vi "Main.vi"() -> ()   [LabVIEW 2019, in "Chat Window.lvlib"]
doc: "This template is based off of the Queued Message Handler design pattern and the Queued Message Handler project template that ships with LabVIEW.\n\nThe main difference is that the queue is private to this module and communication between modules is performed via Broadcast and Request events.\n\nRequest events are wrapped in public API methods and are handled in the Event Handling Loop (EHL) of this VI. Any module can register for Broadcast events sent by this module. The EHL generates messages based on user interface actions.\n\nThe Message Handling Loop (MHL) processes messages generated by the EHL, or by other messages. The messages are string values, so new messages can be added easily to the Message Cases case structure in the MHL. Each message cluster can also provide an optional value for Message Data, which is a variant that can be converted to whatever message-specific data is required.\n_____\nBased on Delacor QMH Project Template 4.2.1.64."
uses:
  Chat Window.lvlib
  <vilib>/Delacor/Delacor QMH/Libraries/Cloneable Module Admin_class/Delacor_lib_QMH_Cloneable Module Admin.lvclass
  C:/Program Files (x86)/National Instruments/LabVIEW 2019/vi.lib/Delacor/Delacor QMH/Libraries/Module Admin_class/Delacor_lib_QMH_Module Admin.lvclass
  Module Data--cluster.ctl
  <vilib>/Delacor/Delacor QMH/Libraries/Message Queue_class/Delacor_lib_QMH_Message Queue.lvclass/Delacor_lib_QMH_Message Queue.ctl
  <vilib>/Delacor/Delacor QMH/Libraries/Cloneable Module Admin_class/Delacor_lib_QMH_Cloneable Module Admin.lvclass/Delacor_lib_QMH_Cloneable Module Admin.ctl
  Stop Argument--cluster.ctl
  New Message Argument--cluster.ctl
  Update Ring Argument--cluster.ctl
  <vilib>/Utility/miscctls.llb/LVPointTypeDef.ctl
  <vilib>/Delacor/Delacor QMH/Libraries/Module Admin_class/Delacor_lib_QMH_Module Admin.lvclass/Delacor_lib_QMH_Module Admin.ctl
  <vilib>/Delacor/Delacor QMH/Libraries/Message Queue_class/Delacor_lib_QMH_Enqueue Message (Single).vi
  <vilib>/Delacor/Delacor QMH/Libraries/Cloneable Module Admin_class/Delacor_lib_QMH_Get Module ID.vi
  <vilib>/Delacor/Delacor QMH/Libraries/Module Admin_class/Delacor_lib_QMH_Get External Launch.vi
  <vilib>/Utility/error.llb/Error Cluster From Error Code.vi
  <vilib>/ErrorRing/Error Ring.xnode
  <vilib>/Delacor/Delacor QMH/Libraries/Message Queue_class/Delacor_lib_QMH_Message Queue.lvclass
  Clone Registration/Clone Registration.lvlib
panel:
  in  "Chat Window Selection":i32(ring) items=["All"=-1]
  in  "Send":bool
  in  "Messages Out":string
  out "Messages In":string
  in  "Simulate MHL Error":bool
  in  "Simulate EHL Error":bool
  out "error out":errorcluster
  in  "Module Admin":refnum<class "Delacor_lib_QMH_Cloneable Module Admin.lvclass">
  out "Status":string
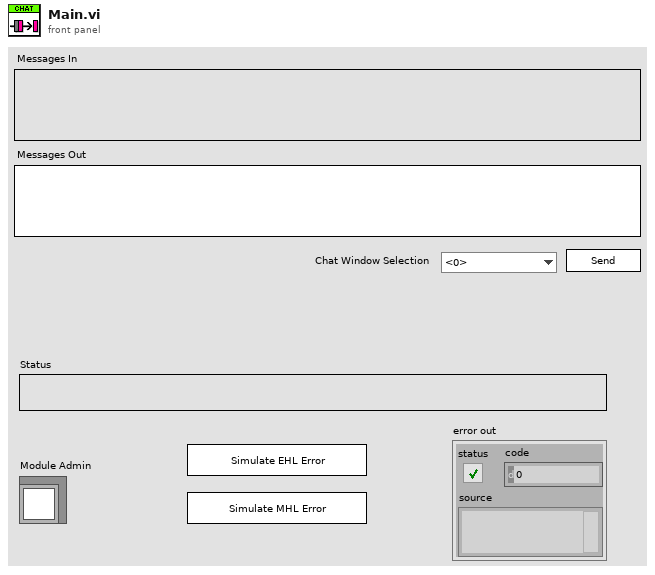
[diagram p1: front panel]
types:
  T1 = typedef "Chat Window.lvlib/Request Events--cluster.ctl" = cluster{"Stop Module":refnum<user-event>, "Show Panel":refnum<user-event>, "Hide Panel":refnum<user-event>, "Show Diagram":refnum<user-event>, "Get Module Execution Status":refnum<user-event>, "New Message":refnum<user-event>, "Update Ring":refnum<user-event>}
  T2 = typedef "Chat Window.lvlib/Module Data--cluster.ctl" = cluster{"Status":string}
  T3 = enum32{"invalid lock state", "Not Locked", "Locked (No Password)", "Password-protected"}
  T4 = typedef "Chat Window.lvlib/Stop Argument--cluster.ctl" = cluster{"Module ID":i32, "Origin":string, "Exit via Stop Module Req?":bool, "Wait for Module to stop?":bool}
  T5 = typedef "Chat Window.lvlib/New Message Argument--cluster.ctl" = cluster{"Module ID":i32, "Chat Message":string}
  T6 = typedef "Chat Window.lvlib/Update Ring Argument--cluster.ctl" = cluster{"Module ID":i32, "Boolean":bool}
  T7 = typedef "LVPointTypeDef.ctl" = cluster{"Horizontal":i16, "Vertical":i16}
  T8 = enum32{"Invalid", "Standard", "Closed", "Hidden", "Minimized", "Maximized"}
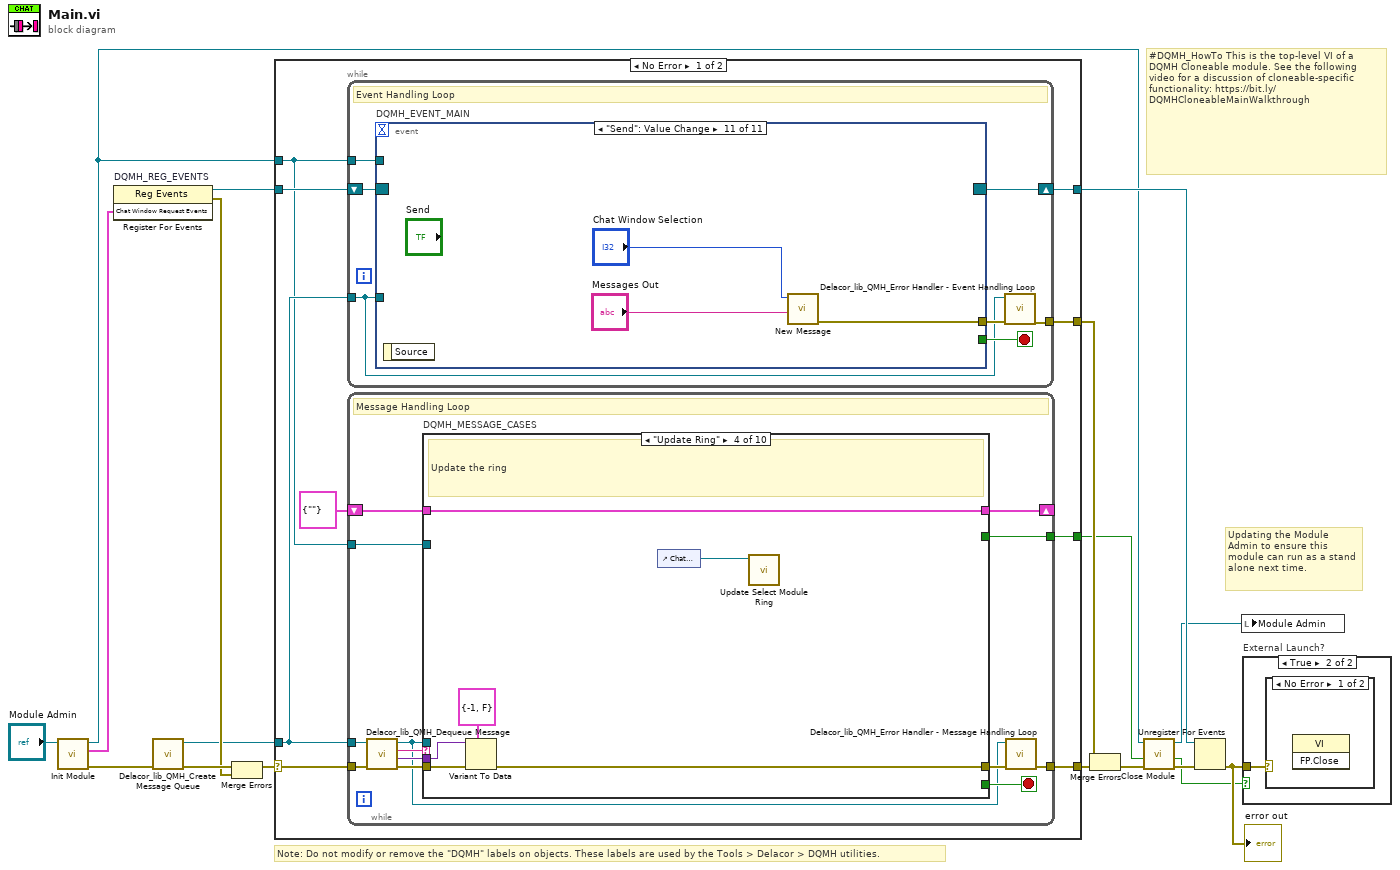
[diagram p0: block diagram]
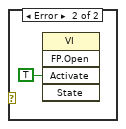
[diagram p3: hidden frame]
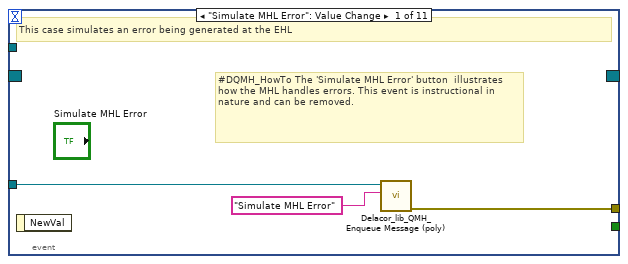
[diagram p4: hidden frame]
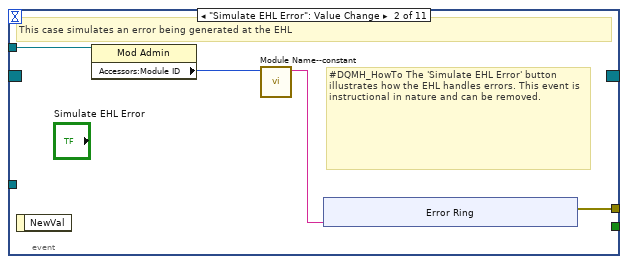
[diagram p5: hidden frame]
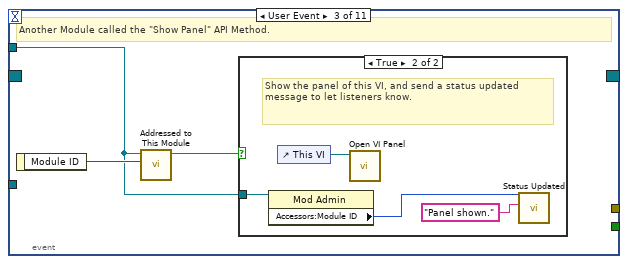
[diagram p6: hidden frame]
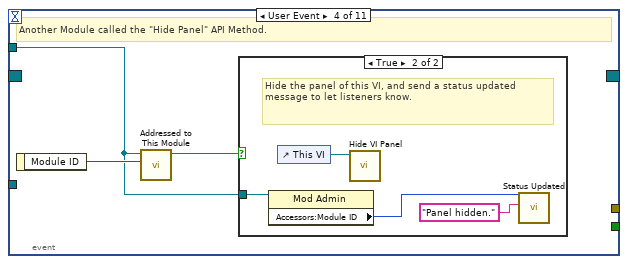
[diagram p8: hidden frame]
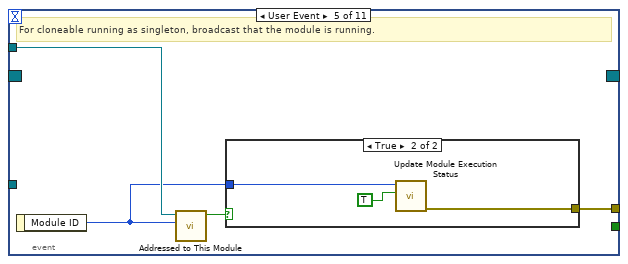
[diagram p10: hidden frame]
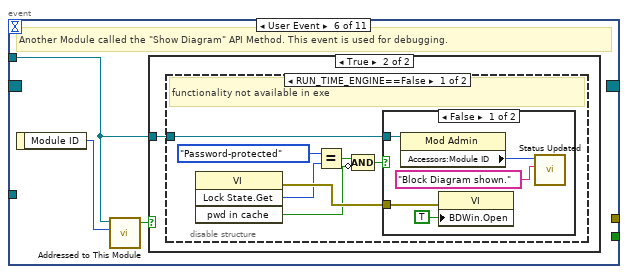
[diagram p12: hidden frame]
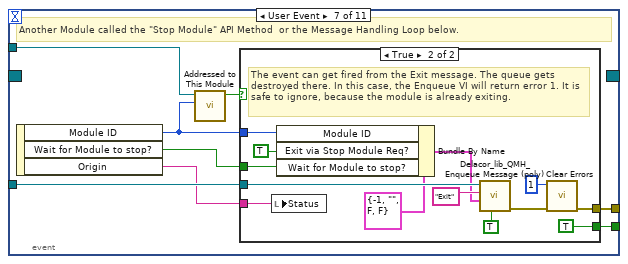
[diagram p16: hidden frame]
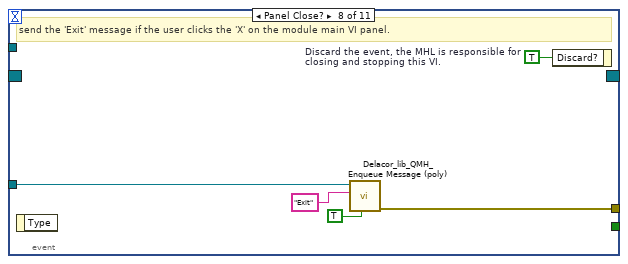
[diagram p18: hidden frame]
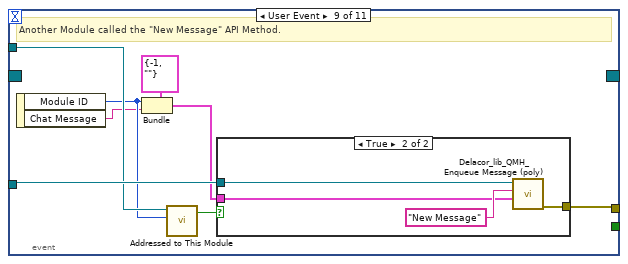
[diagram p19: hidden frame]
diagram:
  # "#DQMH_HowTo This is the top-level VI of a DQMH Cloneable module. See the following video for a discussion of cloneable-specific functionality: https://bit.ly/DQMHCloneableMainWalkthrough"
  # "Note: Do not modify or remove the \"DQMH\" labels on objects. These labels are used by the Tools > Delacor > DQMH utilities."
  # "Updating the Module Admin to ensure this module can run as a stand alone next time."
  n1 = call "Init Module.vi"("Cloneable Module Admin in"="Module Admin") -> ("error out"=w15:errorcluster, "Chat Window Request Events"=w7:T1, "Cloneable Module Admin out"=w4:refnum<class "Delacor_lib_QMH_Cloneable Module Admin.lvclass">)  [unwired: 8 in]
  n2 = register-events "DQMH_REG_EVENTS"(w7) -> (reference out=w8:refnum<event-registration>, error out=w10:errorcluster)  [unwired: 2 in]
  n3 = call <vilib>:"Delacor_lib_QMH_Create Message Queue.vi"("error in (no error)"=w15) -> ("error out"=w12:errorcluster, "Message Queue"=w6:refnum<class "Delacor_lib_QMH_Message Queue.lvclass">)  [unwired: 9 in]
  n4 = Merge Errors(w12, w10) -> (w11:errorcluster)
  n5 = case shown="No Error" w11 {
    selector: w11 -> [w25 w264]
    tunnel: [w27 w264] -> w16
    tunnel: [w24 w263] -> w9
    tunnel: w8 -> [w22 w263]
    tunnel: w6 -> [w21 _]
    tunnel: [w26 _] -> w17
    tunnel: w4 -> [w20 w259]
    tunnel: [w19 _] -> w2
    frame No Error {
      n6 = while {
        tunnel: w21 -> [w28]
        shift-right: [w31] -> w24
        shift-left: w22 -> [w32]
        tunnel: [w33] -> w26
        tunnel: w20 -> [w29]
        stop <- w30 stop-if-true
        # "Event Handling Loop"
        n7 = event "DQMH_EVENT_MAIN" shown="[10] \"Send\": Value Change" {
          selector: w32 -> [_ _ _ _ _ _ _ _ _ _ _]
          dyn-events: [_ _ _ _ _ _ _ _ _ _ _] -> w31
          timeout: _ -> [_ _ _ _ _ _ _ _ _ _ _]
          tunnel: [_ _ _ _ _ _ w89 _ _ _ _] -> w30
          tunnel: w28 -> [w36 _ _ _ _ _ w92 w109 w119 w131 _]
          tunnel: [w37 w41 _ _ w66 _ w93 w111 w112 w124 w136] -> w34
          tunnel: w29 -> [_ w40 w49 w56 w64 w70 w91 _ w117 w129 _]
          event "Simulate MHL Error": Value Change {
            # "#DQMH_HowTo The 'Simulate MHL Error' button  illustrates how the MHL handles errors. This event is instructional in nature and can be removed."
            # "This case simulates an error being generated at the EHL"
            n8 = event-data() -> ()  [unwired: 1 in, 1 out]
            n9 = call-poly <vilib>:"Delacor_lib_QMH_Enqueue Message (poly).vi"("Message"="Simulate MHL Error", "Message Queue in"=w36) -> ("error out"=w37:errorcluster)  [unwired: 8 in, 1 out]
          }
          event "Simulate EHL Error": Value Change {
            # "#DQMH_HowTo The 'Simulate EHL Error' button  illustrates how the EHL handles errors. This event is instructional in nature and can be removed."
            # "This case simulates an error being generated at the EHL"
            n10 = event-data() -> ()  [unwired: 1 in, 1 out]
            n11 = property class="Mod Admin"(reference=w40) -> ("Accessors:Module ID"=w39:i32)  [unwired: 1 in, 2 out]
            n12 = call "Module Name--constant.vi"("Module ID"=w39) -> ("Module Name"=w38:string)  [unwired: 10 in]
            n13 = xnode "Error Ring"("parameter 0"=w38) -> ("error out"=w41:errorcluster)
          }
          event User Event {
            # "Another Module called the \"Show Panel\" API Method."
            n14 = event-data() -> ("Module ID"=w50:i32)  [unwired: 1 in]
            n15 = call "Addressed to This Module.vi"("Module ID from Argument"=w50, "Module Admin"=w49) -> ("Addressed to this instance?"=w51:bool)  [unwired: 8 in, 1 out]
            n16 = case shown="True" w51 {
              tunnel: w49 -> [_ w53]
              frame False {
              }
              frame True {
                # "Show the panel of this VI, and send a status updated message to let listeners know."
                n17 = property class="Mod Admin"(reference=w53) -> ("Accessors:Module ID"=w52:i32)  [unwired: 1 in, 2 out]
                n18 = control-ref of="This VI"() -> (w55:refnum<vi>)
                n19 = call "Open VI Panel.vi"("VI"=w55) -> ()  [unwired: 10 in, 1 out]
                n20 = call "Status Updated.vi"("Status"="Panel shown." ("format string"), "Module ID"=w52) -> ()  [unwired: 9 in, 1 out]
              }
            }
          }
          event User Event {
            # "Another Module called the \"Hide Panel\" API Method."
            n21 = event-data() -> ("Module ID"=w57:i32)  [unwired: 1 in]
            n22 = call "Addressed to This Module.vi"("Module ID from Argument"=w57, "Module Admin"=w56) -> ("Addressed to this instance?"=w58:bool)  [unwired: 8 in, 1 out]
            n23 = case shown="True" w58 {
              tunnel: w56 -> [_ w60]
              frame False {
              }
              frame True {
                # "Hide the panel of this VI, and send a status updated message to let listeners know."
                n24 = property class="Mod Admin"(reference=w60) -> ("Accessors:Module ID"=w59:i32)  [unwired: 1 in, 2 out]
                n25 = control-ref of="This VI"() -> (w62:refnum<vi>)
                n26 = call "Hide VI Panel.vi"("VI"=w62) -> ()  [unwired: 10 in, 1 out]
                n27 = call "Status Updated.vi"("Status"="Panel hidden." ("format string"), "Module ID"=w59) -> ()  [unwired: 9 in, 1 out]
              }
            }
          }
          event User Event {
            # "For cloneable running as singleton, broadcast that the module is running."
            n28 = event-data() -> ("Module ID"=w63:i32)  [unwired: 1 in]
            n29 = call "Addressed to This Module.vi"("Module ID from Argument"=w63, "Module Admin"=w64) -> ("Addressed to this instance?"=w65:bool)  [unwired: 8 in, 1 out]
            n30 = case shown="True" w65 {
              tunnel: [_ w69] -> w66
              tunnel: w63 -> [_ w68]
              frame False {
              }
              frame True {
                n31 = call "Update Module Execution Status.vi"("Running?"=TRUE, "Module ID"=w68) -> ("error out"=w69:errorcluster)  [unwired: 9 in]
              }
            }
          }
          event User Event {
            # "Another Module called the \"Show Diagram\" API Method. This event is used for debugging."
            n32 = event-data() -> ("Module ID"=w71:i32)  [unwired: 1 in]
            n33 = call "Addressed to This Module.vi"("Module ID from Argument"=w71, "Module Admin"=w70) -> ("Addressed to this instance?"=w72:bool)  [unwired: 8 in, 1 out]
            n34 = case shown="True" w72 {
              tunnel: w70 -> [_ w73]
              frame False {
              }
              frame True {
                n35 = disable-structure shown="RUN_TIME_ENGINE==False" {
                  disable-tunnel: w73 -> [w74 _]
                  frame condition #0 (active) {
                    # "functionality not available in exe"
                    n36 = invoke class="VI" method="Lock State.Get"() -> (error out=w80:errorcluster, "Get Lock State"=w79:T3, "pwd in cache"=w76:bool)  [unwired: 4 in, 1 out]
                    n37 = Equal?(x=T3."Password-protected", y=w79) -> (x = y?=w77:bool)
                    n38 = Compound Arithmetic op=AND(w77, invert w76) -> (w75:bool)
                    n39 = case shown="False" w75 {
                      tunnel: w80 -> [w85 _]
                      tunnel: w74 -> [w82 _]
                      frame False {
                        n40 = property class="Mod Admin"(reference=w82) -> ("Accessors:Module ID"=w81:i32)  [unwired: 1 in, 2 out]
                        n41 = property class="VI"(error in=w85, "BDWin.Open"=TRUE ("Block Diagram Window:Open")) -> ()  [unwired: 1 in, 2 out]
                        n42 = call "Status Updated.vi"("Status"="Block Diagram shown." ("format string"), "Module ID"=w81) -> ()  [unwired: 9 in, 1 out]
                      }
                      frame True {
                        # "Password-protected VI, and the password is not in the cache. Do not show the diagram."
                      }
                    }
                  }
                  frame condition #1 {
                  }
                }
              }
            }
          }
          event User Event {
            # "Another Module called the \"Stop Module\" API Method  or the Message Handling Loop below."
            n43 = event-data() -> ("Module ID"=w87:i32, "Wait for Module to stop?"=w88:bool, "Origin"=w86:string)  [unwired: 1 in]
            n44 = call "Addressed to This Module.vi"("Module ID from Argument"=w87, "Module Admin"=w91) -> ("Addressed to this instance?"=w90:bool)  [unwired: 8 in, 1 out]
            n45 = case shown="True" w90 {
              tunnel: [_ w105] -> w93
              tunnel: w92 -> [_ w101]
              tunnel: [_ TRUE] -> w89
              tunnel: w88 -> [_ w96]
              tunnel: w87 -> [_ w98]
              tunnel: w86 -> [_ w94]
              frame False {
              }
              frame True {
                # "The event can get fired from the Exit message. The queue gets destroyed there. In this case, the Enqueue VI will return error 1. It is safe to ignore, because the module is already exiting."
                n46 = local write "Status"(w94) -> ()
                n47 = Bundle By Name(cluster=T4 {"Module ID"=-1, "Origin"="", "Exit via Stop Module Req?"=FALSE, "Wait for Module to stop?"=FALSE} ("Stop Argument"), "Module ID"=w98, "Exit via Stop Module Req?"=TRUE, "Wait for Module to stop?"=w96) -> (w95:T4)
                n48 = call-poly <vilib>:"Delacor_lib_QMH_Enqueue Message (poly).vi"("Priority Message? (F)"=TRUE, "Message Data"=w95, "Message"="Exit", "Message Queue in"=w101) -> ("error out"=w106:errorcluster)  [unwired: 6 in, 1 out]
                n49 = call <vilib>:"Clear Errors.vi"("error in (no error)"=w106, "specific error code to clear (0: all)"=1) -> ("error out"=w105:errorcluster)  [unwired: 4 in, 1 out]
              }
            }
          }
          event Panel Close? {
            w110 = TRUE  # Discard the event, the MHL is responsible for closing and stopping this VI.
            # "send the 'Exit' message if the user clicks the 'X' on the module main VI panel."
            n50 = event-data() -> ()  [unwired: 1 in, 1 out]
            n51 = call-poly <vilib>:"Delacor_lib_QMH_Enqueue Message (poly).vi"("Priority Message? (F)"=TRUE, "Message"="Exit", "Message Queue in"=w109) -> ("error out"=w111:errorcluster)  [unwired: 7 in, 1 out]
            n52 = event-data("Discard?"=w110) -> ()  [unwired: 1 in, 1 out]
          }
          event User Event {
            # "Another Module called the \"New Message\" API Method."
            n53 = event-data() -> ("Module ID"=w114:i32, "Chat Message"=w113:string)  [unwired: 1 in]
            n54 = Bundle(cluster=T5 {"Module ID"=-1, "Chat Message"=""} ("New Message Argument"), "Module ID"=w114, "Chat Message"=w113) -> (w115:T5)
            n55 = call "Addressed to This Module.vi"("Module ID from Argument"=w114, "Module Admin"=w117) -> ("Addressed to this instance?"=w118:bool)  [unwired: 8 in, 1 out]
            n56 = case shown="True" w118 {
              tunnel: w119 -> [_ w123]
              tunnel: w115 -> [_ w121]
              tunnel: [_ w120] -> w112
              frame False {
              }
              frame True {
                n57 = call-poly <vilib>:"Delacor_lib_QMH_Enqueue Message (poly).vi"("Message Data"=w121, "Message"="New Message", "Message Queue in"=w123) -> ("error out"=w120:errorcluster)  [unwired: 7 in, 1 out]
              }
            }
          }
          event User Event {
            # "Another Module called the \"Update Ring\" API Method."
            n58 = event-data() -> ("Module ID"=w126:i32, "Boolean"=w125:bool)  [unwired: 1 in]
            n59 = Bundle(cluster=T6 {"Module ID"=-1, "Boolean"=FALSE} ("Update Ring Argument"), "Module ID"=w126, "Boolean"=w125) -> (w127:T6)
            n60 = call "Addressed to This Module.vi"("Module ID from Argument"=w126, "Module Admin"=w129) -> ("Addressed to this instance?"=w130:bool)  [unwired: 8 in, 1 out]
            n61 = case shown="True" w130 {
              tunnel: w131 -> [_ w135]
              tunnel: w127 -> [_ w133]
              tunnel: [_ w132] -> w124
              frame False {
              }
              frame True {
                n62 = call-poly <vilib>:"Delacor_lib_QMH_Enqueue Message (poly).vi"("Message Data"=w133, "Message"="Update Ring", "Message Queue in"=w135) -> ("error out"=w132:errorcluster)  [unwired: 7 in, 1 out]
              }
            }
          }
          event "Send": Value Change {
            n63 = event-data() -> ()  [unwired: 1 in, 1 out]
            n64 = call "New Message.vi"("Chat Message"="Messages Out", "Module ID"="Chat Window Selection") -> ("error out"=w136:errorcluster)  [unwired: 9 in]
          }
        }
        n65 = call-dynamic "Delacor_lib_QMH_Error Handler - Event Handling Loop.vi"("error in (no error)"=w34, "Message Queue in"=w28) -> ("dup error in"=w33:errorcluster)  [unwired: 8 in, 1 out]
      }
      n66 = while {
        tunnel: w21 -> [w142]
        shift-right: [w146] -> _
        shift-left: T2 {"Status"=""} ("Data Cluster") -> [w147]
        tunnel: w25 -> [w150]
        tunnel: [w148] -> w27
        tunnel: w20 -> [w140]
        tunnel: [w139] -> w19
        stop <- w145 stop-if-true
        # "Message Handling Loop"
        n67 = call-dynamic "Delacor_lib_QMH_Dequeue Message.vi"("error in (no error)"=w150, "Message Queue in"=w142) -> ("error out"=w149:errorcluster, "Message Data"=w143:variant, "Message"=w144:string, "Message Queue out"=w141:refnum<class "Delacor_lib_QMH_Message Queue.lvclass">)  [unwired: 6 in]
        n68 = case "DQMH_MESSAGE_CASES" shown="\"Update Ring\"" w144 {
          selector: w144 -> [_ _ _ _ _ _ _ _ _ w244]
          tunnel: w141 -> [_ _ _ _ _ _ w194 _ w234 _]
          tunnel: w149 -> [w171 w175 w182 w188 w191 w193 w204 w217 w240 w246]
          tunnel: [w169 w175 w180 w186 w190 w193 w200 w216 w237 w247] -> w151
          tunnel: w147 -> [w162 w174 w181 w187 w189 w192 w199 w214 w233 w245]
          tunnel: [w161 w174 w181 w187 w189 w192 w199 w214 w233 w245] -> w146
          tunnel: [_ _ _ _ _ _ _ _ w232 _] -> w145
          tunnel: w143 -> [_ _ w179 w185 _ _ w198 _ w230 _]
          tunnel: w140 -> [w156 _ _ _ _ _ w197 w212 w226 w242]
          tunnel: [_ _ _ _ _ _ _ _ w228 _] -> w139
          frame "Initialize" {
            w153 = "Initial Message" ("Initial Message")
            # "Initialize - Any operation that needs to be done before the module can receive messages. Synchronize Caller Events.vi will inform Start Module.vi that the module has launched and is ready to receive messages. Module Did Init.vi will broadcast that the module initialized."
            n69 = call "Synchronize Caller Events.vi"("error in (no error)"=w171, "Module Admin"=w156) -> ("error out"=w170:errorcluster, "Module Admin out"=w155:refnum<class "Delacor_lib_QMH_Cloneable Module Admin.lvclass">)  [unwired: 8 in]
            n70 = control-ref of="Chat Window Selection"() -> (w152:refnum<vi>)
            n71 = property class="Mod Admin"(reference=w155) -> ("Accessors:Module ID"=w158:i32, "Accessors:External Launch"=w157:bool)  [unwired: 1 in, 2 out]
            n72 = call "Init Select Module Ring.vi"("Select Module Ring Ref"=w152) -> ()  [unwired: 8 in, 3 out]
            n73 = call "Module Name--constant.vi"("Module ID"=w158) -> ("Module Name"=w166:string)  [unwired: 10 in]
            n74 = property class="VI"("Front Panel.Title"=w166) -> (reference out=w168:refnum<vi>, error out=w173:errorcluster)  [unwired: 2 in]
            n75 = Select(t=T8."Hidden" ("State"), s=w157, f=T8."Standard" ("State")) -> (s? t:f=w163:T8)
            n76 = invoke class="VI" method="FP.Open"(reference=w168, error in=w173, "State"=w163) -> (reference out=w167:refnum<vi>, error out=w172:errorcluster)  [unwired: 2 in, 3 out]
            n77 = call "Module Name--constant.vi"("Module ID"=w158) -> ("Module Name"=w159:string)  [unwired: 10 in]
            n78 = Bundle By Name(cluster=w162, "Status"=w153) -> (w161:T2)
            n79 = invoke class="VI" method="FP.Center"(reference=w167, error in=w172) -> ()  [unwired: 1 in, 3 out]
            n80 = property on="Pane" class="Pane"("Origin"=T7 {"Horizontal"=0, "Vertical"=0}) -> ()  [unwired: 2 in, 2 out]
            n81 = call "Module Did Init.vi"("error in (no error)"=w170, "Initialized?"=TRUE, "Origin"=w159, "Module ID"=w158) -> ("error out"=w169:errorcluster)  [unwired: 7 in]
            "Status" <- w153
          }
          frame "--- Module Specific ---" {
            # "Separator -- The following cases handle messages specific to this Module."
          }
          frame "New Message" {
            # "A new message was sent to this chat window."
            n82 = Variant To Data(error in=w182, type=T5 {"Module ID"=-1, "Chat Message"=""} ("New Message Argument"), Variant=w179) -> (data=w177:T5, error out=w180:errorcluster)
            n83 = Unbundle By Name(w177) -> ("Chat Message"=→"Messages In":string)  [unwired: 1 out]
          }
          frame "Update Ring" {
            # "Update the ring"
            n84 = Variant To Data(error in=w188, type=T6 {"Module ID"=-1, "Boolean"=FALSE} ("Update Ring Argument"), Variant=w185) -> (error out=w186:errorcluster)  [unwired: 1 out]
            n85 = control-ref of="Chat Window Selection"() -> (w183:refnum<vi>)
            n86 = call "Update Select Module Ring.vi"("Select Module Ring Ref"=w183) -> ()  [unwired: 8 in, 3 out]
          }
          frame "---Copy This Frame---" {
            # "Duplicate this frame when creating new messages.  Change this comment in the duplicated frame to describe this message."
            n87 = Merge Errors(w191) -> (w190:errorcluster)
          }
          frame "--- Exit and Error Handling---" {
            # "Separator - the following cases handle errors and exit messages."
          }
          frame "Error" {
            # "#CodeRecommended - If you ever change the name of this \"Error\" message, you'll need to update the name in the Check Loop Error.vi as well."
            # "#CodeRecommended - If the module is running in standalone mode (External Launch = FALSE), this code will pop up an error dialog and call the 'Exit' message if an error occurs. Add more fine-grained error handling here."
            # "Error - Check the error message data and respond accordingly. This message is sent by the \"Error Handler\" VIs at the end of each loop in this application."
            n88 = property class="Mod Admin"(reference=w197) -> ("Accessors:External Launch"=w195:bool, "Accessors:Module ID"=w196:i32)  [unwired: 1 in, 2 out]
            n89 = Variant To Data(error in=w204, type=errorcluster {"status"=FALSE, "code"=0, "source"=""} ("error constant"), Variant=w198) -> (data=w205:errorcluster, error out=w202:errorcluster)
            n90 = call "Error Reported.vi"("Error"=w205, "Module ID"=w196) -> ()  [unwired: 9 in, 1 out]
            n91 = case shown="False" w195 {
              tunnel: [w210 _] -> w201
              tunnel: w194 -> [w208 _]
              tunnel: w205 -> [w209 _]
              frame False {
                # "If the module is running standalone, then pop up an error dialog and call the \"Exit\" message."
                n92 = call <vilib>:"Simple Error Handler.vi"("error in (no error)"=w209) -> ()  [unwired: 4 in, 5 out]
                n93 = call-poly <vilib>:"Delacor_lib_QMH_Enqueue Message (poly).vi"("Priority Message? (F)"=TRUE, "Message"="Exit", "Message Queue in"=w208) -> ("error out"=w210:errorcluster)  [unwired: 7 in, 1 out]
              }
              frame True {
                # "If the module was launched externally, calling the Error Reported broadcast VI is the only action performed by the \"Error\" message. The module's caller can then process the error appropriately."
              }
            }
            n94 = Merge Errors(w202, w201) -> (w200:errorcluster)
            n95 = local write "error out"(w200) -> ()
          }
          frame "Simulate MHL Error" {
            # "#DQMH_HowTo The 'Simulate MHL Error' button  illustrates how the MHL handles errors. This event is instructional in nature and can be removed."
            # "Simulate an error occurring at the MHL"
            n96 = property class="Mod Admin"(reference=w212) -> ("Accessors:Module ID"=w213:i32)  [unwired: 1 in, 2 out]
            n97 = call "Module Name--constant.vi"("Module ID"=w213) -> ("Module Name"=w211:string)  [unwired: 10 in]
            n98 = xnode "Error Ring"("parameter 0"=w211) -> ("error out"=w215:errorcluster)
            n99 = Merge Errors(w217, w215) -> (w216:errorcluster)
          }
          frame "Exit" {
            w231 = 91  # 91: not all Exit messages will have an argument
            w232 = TRUE  # Stop the VI
            # "Release the message queue reference"
            # "#CodeNeeded - Add any required cleanup code here."
            # "Exit - Exit the application."
            n100 = Variant To Data(error in=w240, type=T4 {"Module ID"=-1, "Origin"="", "Exit via Stop Module Req?"=FALSE, "Wait for Module to stop?"=FALSE} ("Stop Argument"), Variant=w230) -> (data=w227:T4, error out=w235:errorcluster)
            n101 = call <vilib>:"Clear Errors.vi"("error in (no error)"=w235, "specific error code to clear (0: all)"=w231) -> ("error out"=w239:errorcluster)  [unwired: 4 in, 1 out]
            n102 = control-ref of="This VI"() -> (w225:refnum<vi>)
            n103 = call-dynamic "Delacor_lib_QMH_Release Message Queue.vi"("error in (no error)"=w239, "Message Queue"=w234) -> ("error out"=w238:errorcluster)  [unwired: 9 in]
            n104 = call "Handle Exit.vi"("Stop Argument"=w227, "Module Admin in"=w226, "VI reference"=w225) -> ("error out"=w236:errorcluster, "Wait for Stop?"=w228:bool)  [unwired: 7 in]
            n105 = Merge Errors(w238, w236) -> (w237:errorcluster)
          }
          frame Default {
            # "'Default' case only runs if there is a message that isn't defined in any of the other cases.  Output a programming error."
            n106 = property class="Mod Admin"(reference=w242) -> ("Accessors:Module ID"=w241:i32)  [unwired: 1 in, 2 out]
            n107 = call "Module Name--constant.vi"("Module ID"=w241) -> ("Module Name"=w243:string)  [unwired: 10 in]
            n108 = xnode "Error Ring"("parameter 0"=w244, "parameter 1"=w243) -> ("error out"=w248:errorcluster)
            n109 = Merge Errors(w246, w248) -> (w247:errorcluster)
          }
        }
        n110 = call-dynamic "Delacor_lib_QMH_Error Handler - Message Handling Loop.vi"("error in (no error)"=w151, "Message Queue in"=w141) -> ("dup error in"=w148:errorcluster)  [unwired: 8 in, 1 out]
      }
    }
    frame Error {
      n111 = call "Synchronize Caller Events.vi"("Module Admin"=w259) -> ("Module Admin out"=w258:refnum<class "Delacor_lib_QMH_Cloneable Module Admin.lvclass">)  [unwired: 9 in, 1 out]
      n112 = property class="Mod Admin"(reference=w258) -> ("Accessors:Module ID"=w257:i32)  [unwired: 1 in, 2 out]
      n113 = call "Module Name--constant.vi"("Module ID"=w257) -> ("Module Name"=w262:string)  [unwired: 10 in]
      n114 = call "Remove.vi"("Module ID"=w257) -> ()  [unwired: 9 in, 2 out]
      n115 = Format Into String(format string="An error occurred during initialization. %s is no longer running.", w262) -> (resulting string=w260:string)  [unwired: 2 in, 1 out]
      n116 = call "Error Reported.vi"("Additional Information"=w260, "Error"=w264, "Module ID"=w257) -> ()  [unwired: 8 in, 1 out]
    }
  }
  n117 = Merge Errors(w17, w16) -> (w18:errorcluster)
  n118 = call "Close Module.vi"("error in (no error)"=w18, "Wait for stop?"=w2, "Module Admin in"=w4) -> ("error out"=w14:errorcluster, "External Launch"=w1:bool, "Module Admin out"=w3:refnum<class "Delacor_lib_QMH_Cloneable Module Admin.lvclass">)  [unwired: 6 in]
  n119 = Unregister For Events(event registration refnum=w9, error in=w14) -> (error out=w13:errorcluster)
  "error out" <- w13
  n120 = local write "Module Admin"(w3) -> ()
  n121 = case "External Launch?" shown="True" w1 {
    tunnel: w13 -> [_ w265]
    frame False {
    }
    frame True {
      n122 = case shown="No Error" w265 {
        frame No Error {
          n123 = invoke class="VI" method="FP.Close"() -> ()  [unwired: 3 in, 3 out]
        }
        frame Error {
          n124 = invoke class="VI" method="FP.Open"("Activate"=TRUE ("Activate?")) -> ()  [unwired: 4 in, 5 out]
        }
      }
    }
  }
